vi "IMAQ FPGA CXP Address Generator 6Bit.vi"(0 "Base Address":u8, 1 "Index":u8=1) -> (6 "Address Out":u8)   [LabVIEW 2020]
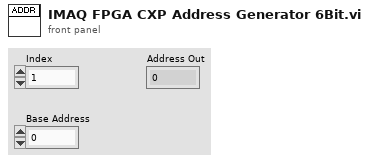
[diagram p1: front panel]
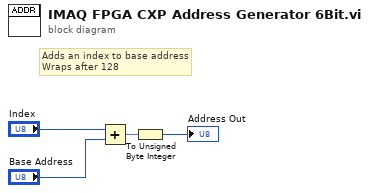
[diagram p0: block diagram]
diagram:
  # "Adds an index to base address\nWraps after 128"
  n1 = Add(x="Index", y="Base Address") -> (x+y=w1:fxp<+,6,6>)
  n2 = To Unsigned Byte Integer(number=w1) -> (unsigned 8bit integer=→"Address Out":u8)
